vi "sub_setBooleanDisplayText.vi"(6 "symbol":string, 9 "selection index":i32, 10 "Enum":enum16{"initialize", "set control value"}(ring), 11 "control references":refnum<vi>[](array[refnum])) -> ()   [LabVIEW 2018]
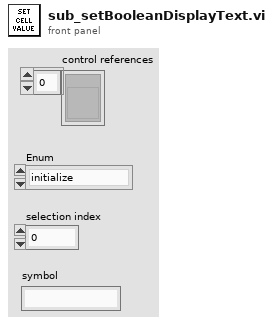
[diagram p1: front panel]
types:
  T1 = enum8{"Enabled", "Disabled", "Disabled and Grayed Out"}
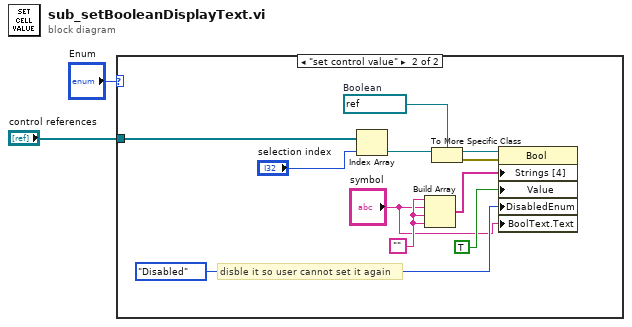
[diagram p0: block diagram]
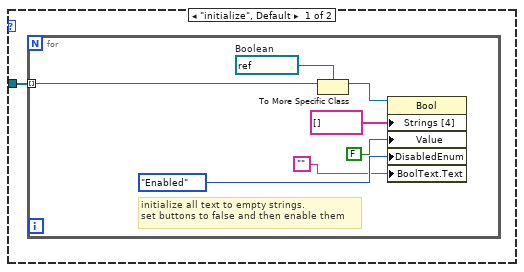
[diagram p2: hidden frame]
diagram:
  n1 = case shown="\"set control value\"" "Enum" {
    tunnel: "control references" -> [w3 w14]
    frame "initialize", Default {
      n2 = for {
        tunnel: w3 -> [w7] mode=indexing
        w6 = refnum<vi> refnum  # Boolean
        # "initialize all text to empty strings.\nset buttons to false and then enable them"
        n3 = To More Specific Class(target class=w6, reference=w7) -> (specific class reference=w5:refnum<vi>)  [unwired: 1 in, 1 out]
        n4 = property class="Bool"(reference=w5, "Strings [4]"=string[] [], "Value"=FALSE, "DisabledEnum"=T1."Enabled" ("Disabled"), "BoolText.Text"="") -> ()  [unwired: 1 in, 2 out]
      }
    }
    frame "set control value" {
      w17 = refnum<vi> refnum  # Boolean
      w19 = ""
      # "disble it so user cannot set it again"
      n5 = Index Array(array=w14, index="selection index") -> (element=w12:refnum<vi>)
      n6 = Build Array(w19, "symbol", w19, w19) -> (w18:string[])
      n7 = To More Specific Class(target class=w17, reference=w12) -> (specific class reference=w16:refnum<vi>, error out=w15:errorcluster)  [unwired: 1 in]
      n8 = property class="Bool"(reference=w16, error in=w15, "Strings [4]"=w18, "Value"=TRUE, "DisabledEnum"=T1."Disabled" ("Disabled"), "BoolText.Text"="symbol") -> ()  [unwired: 2 out]
    }
  }
